vi "ISO 8601 filename.vi"(8 "error in (no error)":errorcluster) -> (0 "error out":errorcluster)   [LabVIEW 2026, in "Tests.lvlib"]
doc: "Unit test (Caraya) for the log file-name builder.\nVerifies a file name is an optional baseName prefix plus an ISO 8601 timestamp with colons removed (so it is valid on Windows and still sorts chronologically), then a normalized extension. Covers the empty-baseName (timestamp-only) form and extension normalization: a leading dot is optional and an empty extension yields no trailing dot.\nPure test: builds names from known inputs and asserts on the returned string. No file I/O, no fixture.\n\nImplements LMBR-T-035, T-036, T-037 -> SRS-035. Assert-level IDs: Test-ID-Assert-Checklist.md."
uses:
  Tests.lvlib
  <vilib>/addons/_JKI Toolkits/Caraya/classes/Assert/Assert Equal Value_Variant.vi
  <vilib>/addons/_JKI Toolkits/Caraya/classes/Assert/Assert True.vi
  <vilib>/addons/_JKI Toolkits/Caraya/classes/Test/Test.lvclass
  src/Lumberjack.lvlib
  <vilib>/addons/_JKI Toolkits/Caraya/classes/Assert/Assert.lvclass
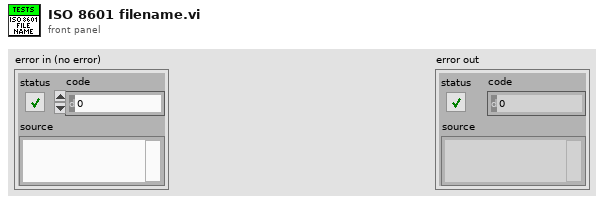
[diagram p1: front panel]
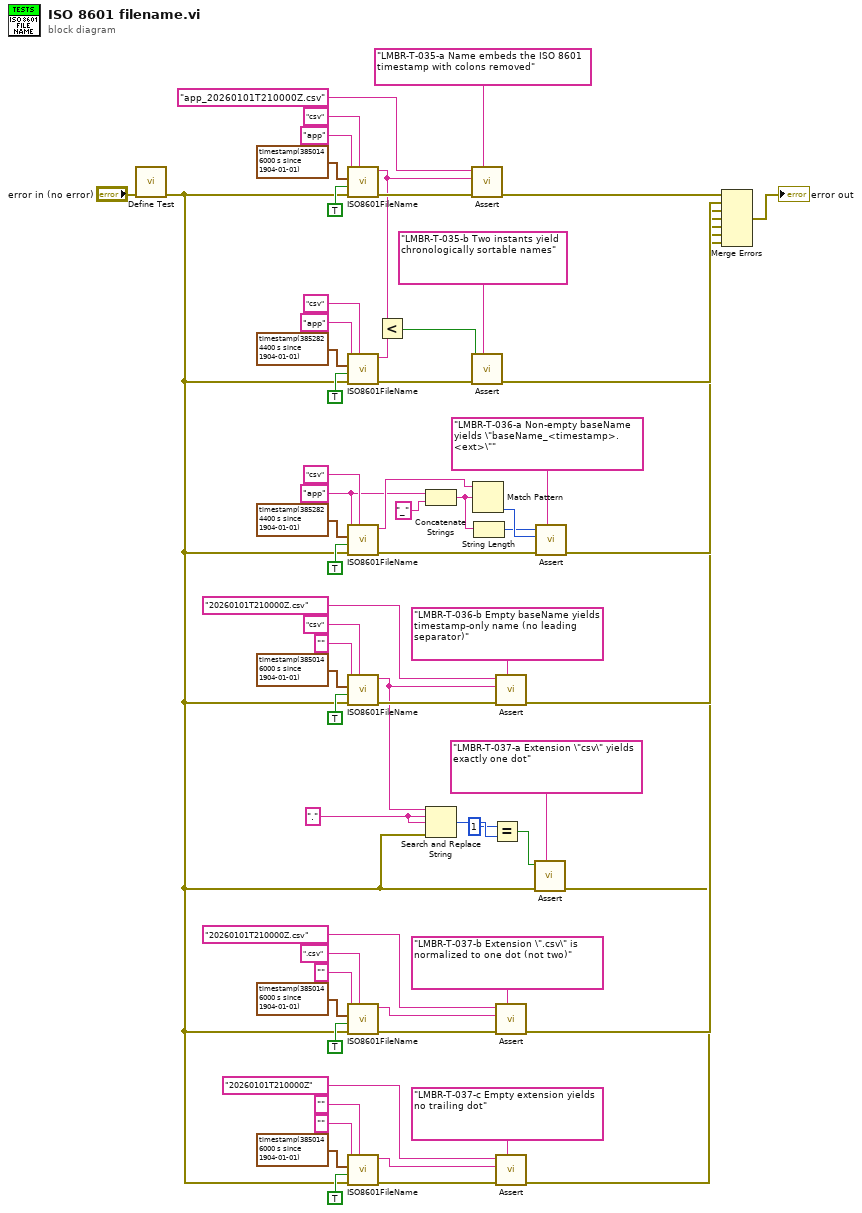
[diagram p0: block diagram]
diagram:
  w25 = "." ("search string")
  w44 = "app" ("BaseName")
  n1 = call <vilib>:"Define Test.vi"("error in (no error)"="error in (no error)") -> ("error out"=w3:errorcluster)  [unwired: 9 in, 1 out]
  n2 = call "ISO8601FileName.vi"("Extension"="csv", "error in (no error)"=w3, "useUTC"=TRUE, "Timestamp"=timestamp(3850146000 s since 1904-01-01), "BaseName"="app") -> ("error out"=w57:errorcluster, "FileName"=w53:string)  [unwired: 5 in]
  n3 = call "ISO8601FileName.vi"("Extension"="csv", "error in (no error)"=w3, "useUTC"=TRUE, "Timestamp"=timestamp(3852824400 s since 1904-01-01), "BaseName"="app") -> ("error out"=w51:errorcluster, "FileName"=w52:string)  [unwired: 5 in]
  n4 = call "ISO8601FileName.vi"("Extension"="csv", "error in (no error)"=w3, "useUTC"=TRUE, "Timestamp"=timestamp(3852824400 s since 1904-01-01), "BaseName"=w44) -> ("error out"=w42:errorcluster, "FileName"=w45:string)  [unwired: 5 in]
  n5 = call "ISO8601FileName.vi"("Extension"="csv", "error in (no error)"=w3, "useUTC"=TRUE, "Timestamp"=timestamp(3850146000 s since 1904-01-01), "BaseName"="") -> ("error out"=w31:errorcluster, "FileName"=w26:string)  [unwired: 5 in]
  n6 = call "ISO8601FileName.vi"("Extension"=".csv", "error in (no error)"=w3, "useUTC"=TRUE, "Timestamp"=timestamp(3850146000 s since 1904-01-01), "BaseName"="") -> ("error out"=w17:errorcluster, "FileName"=w13:string)  [unwired: 5 in]
  n7 = call "ISO8601FileName.vi"("Extension"="", "error in (no error)"=w3, "useUTC"=TRUE, "Timestamp"=timestamp(3850146000 s since 1904-01-01), "BaseName"="") -> ("error out"=w8:errorcluster, "FileName"=w4:string)  [unwired: 5 in]
  n8 = Less?(x=w53, y=w52) -> (x < y?=w50:bool)
  n9 = Concatenate Strings(w44, "_" ("string")) -> (w36:string)
  n10 = Search and Replace String(input string=w26, search string=w25, replace string=w25, error in=w3) -> (number of replacements=w24:i32)  [unwired: 4 in, 3 out]
  n11 = call-poly <vilib>:"Assert.vi"("Label"="LMBR-T-035-a Name embeds the ISO 8601 timestamp with colons removed" ("Extension"), "error in (no error)"=w57, "Actual"=w53, "Expected"="app_20260101T210000Z.csv" ("Extension")) -> ("error out"=w54:errorcluster)  [unwired: 6 in, 1 out]
  n12 = call-poly <vilib>:"Assert.vi"("Label"="LMBR-T-035-b Two instants yield chronologically sortable names" ("Extension"), "error in (no error)"=w51, "True?"=w50) -> ("error out"=w48:errorcluster)  [unwired: 7 in, 1 out]
  n13 = Match Pattern(string=w45, regular expression=w36) -> (offset past match=w37:i32)  [unwired: 1 in, 3 out]
  n14 = String Length(string=w36) -> (length=w35:i32)
  n15 = Equal?(x=1, y=w24) -> (x = y?=w22:bool)
  n16 = call-poly <vilib>:"Assert.vi"("Label"="LMBR-T-036-b Empty baseName yields timestamp-only name (no leading separator)" ("Extension"), "error in (no error)"=w31, "Actual"=w26, "Expected"="20260101T210000Z.csv" ("Extension")) -> ("error out"=w28:errorcluster)  [unwired: 6 in, 1 out]
  n17 = call-poly <vilib>:"Assert.vi"("Label"="LMBR-T-037-b Extension \".csv\" is normalized to one dot (not two)" ("Extension"), "error in (no error)"=w17, "Actual"=w13, "Expected"="20260101T210000Z.csv" ("Extension")) -> ("error out"=w12:errorcluster)  [unwired: 6 in, 1 out]
  n18 = call-poly <vilib>:"Assert.vi"("Label"="LMBR-T-037-c Empty extension yields no trailing dot" ("Extension"), "error in (no error)"=w8, "Actual"=w4, "Expected"="20260101T210000Z" ("Extension")) -> ("error out"=w2:errorcluster)  [unwired: 6 in, 1 out]
  n19 = call-poly <vilib>:"Assert.vi"("Label"="LMBR-T-037-a Extension \"csv\" yields exactly one dot" ("Extension"), "error in (no error)"=w3, "True?"=w22) -> ("error out"=w1:errorcluster)  [unwired: 7 in, 1 out]
  n20 = call-poly <vilib>:"Assert.vi"("Label"="LMBR-T-036-a Non-empty baseName yields \"baseName_<timestamp>.<ext>\"" ("Extension"), "error in (no error)"=w42, "Actual"=w37, "Expected"=w35) -> ("error out"=w40:errorcluster)  [unwired: 6 in, 1 out]
  n21 = Merge Errors(w54, w48, w40, w28, w1, w12, w2) -> (→"error out":errorcluster)
